vi "Key.vi"(6 "Scale":T1=enum."DO", 8 "Key":u8, 9 "Enable":bool) -> (0 "M":fxp<+,32,32>, 4 "Key out":u8)   [LabVIEW 2015]
uses:
  TypeDefs Host/Scales.ctl
panel:
  # "1"
  # "2"
  # "3"
  # "4"
  # "5"
  # "DO\nDO#\nRE\nRE#\nMI\nFA\nFA#\nSOL\nSOL#\nLA\nLA#\nSI"
  # "65,41\n69,30\n73,42\n77,78\n82,41\n87,31\n92,50\n98\n103,83\n110\n116,62\n123,47"
  # "130.82\n138.59\n146.83\n155.56\n164.81\n174.61\n185\n196\n207.65\n220\n233.08\n246.94"
  # "261.63\n277.18\n293.66\n311.13\n329.63\n349.23\n369.99\n392\n415.3\n440\n466.16\n493.88"
  # "523.25\n554.37\n587.33\n622.25\n659.26\n698.46\n739.99\n783.99\n830.61\n880\n932.33\n987.77"
  # "1046.5\n1108.73\n1174.66\n1244.51\n1318.51\n1396.91\n1479.98\n1567.98\n1661.22\n1760\n1864.66\n1975.53\n2093.00"
  # "65,41\n69,30\n73,42\n77,78\n82,41\n87,31\n92,50\n98\n103,83\n110\n116,62\n123,47"
  # "130.82\n138.59\n3941437,800448\n155.56\n4424084,750336\n174.61\n4966055,936\n5261334,9376\n207.65\n5905580,032\n233.08\n6628745,150464"
  # "261.63\n7440493,969408\n7882875,600896\n311.13\n8848437,936128\n349.23\n9931843,436544\n10522669,8752\n415.3\n11811160,064\n466.16\n13257490,300928"
  # "523.25\n14881256,374272\n15766019,637248\n622.25\n659.26\n698.46\n739.99\n783.99\n830.61\n880\n932.33\n987.77"
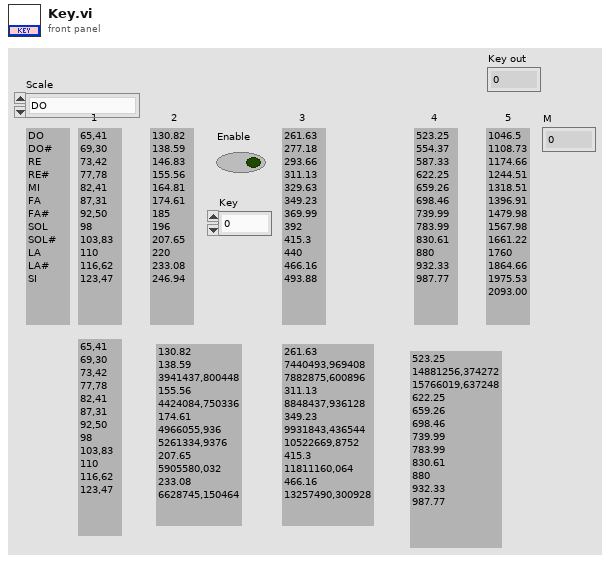
[diagram p1: front panel]
types:
  T1 = typedef "Scales.ctl" = enum16{"ALL", "DO", "RE"}
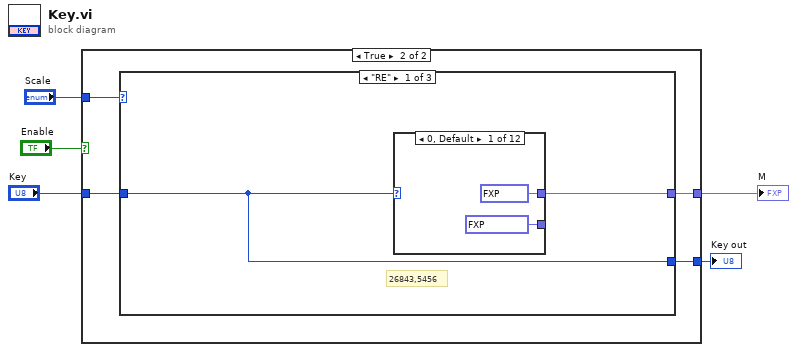
[diagram p0: block diagram]
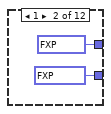
[diagram p3: hidden frame]
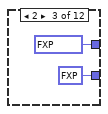
[diagram p4: hidden frame]
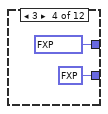
[diagram p5: hidden frame]
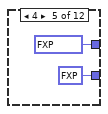
[diagram p6: hidden frame]
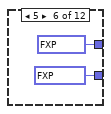
[diagram p7: hidden frame]
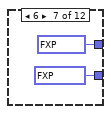
[diagram p8: hidden frame]
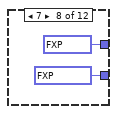
[diagram p9: hidden frame]
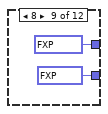
[diagram p10: hidden frame]
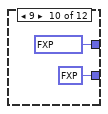
[diagram p11: hidden frame]
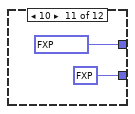
[diagram p12: hidden frame]
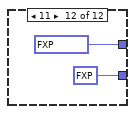
[diagram p13: hidden frame]
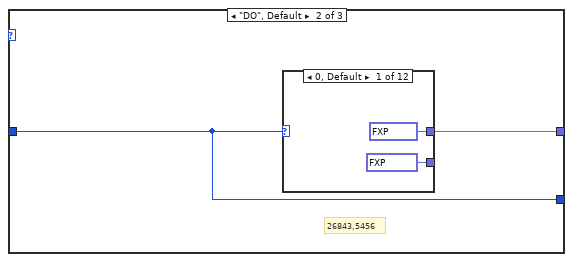
[diagram p14: hidden frame]
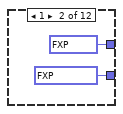
[diagram p15: hidden frame]
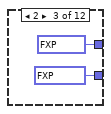
[diagram p16: hidden frame]
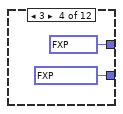
[diagram p17: hidden frame]
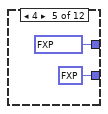
[diagram p18: hidden frame]
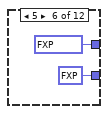
[diagram p19: hidden frame]
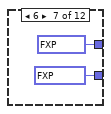
[diagram p20: hidden frame]
diagram:
  n1 = case shown="True" "Enable" {
    tunnel: "Key" -> [_ w9]
    tunnel: "Scale" -> [_ w8]
    tunnel: [_ w7] -> w3
    tunnel: [_ w6] -> w1
    frame False {
    }
    frame True {
      n2 = case shown="\"RE\"" w8 {
        tunnel: w9 -> [w10 w36 w65]
        tunnel: [w11 w37 w68] -> w7
        tunnel: [w10 w36 _] -> w6
        frame "RE" {
          # "26843,5456"
          n3 = case shown="0, Default" w10 {
            tunnel: [fxp<+,16,10> 146.828125 ("Fout 2") fxp<+,16,10> 164.8125 ("Fout 2") fxp<+,16,10> 185.0 ("Fout 2") fxp<+,16,10> 196.0 ("Fout 2") fxp<+,16,10> 220.0 ("Fout 2") fxp<+,16,10> 246.9375 ("Fout 2") fxp<+,16,10> 277.1875 ("Fout 2") fxp<+,16,10> 293.65625 ("Fout 2") fxp<+,16,10> 329.625 ("Fout 2") fxp<+,16,10> 370.0 ("Fout 2") fxp<+,16,10> 392.0 ("Fout 2") fxp<+,16,10> 440.0 ("Fout 2")] -> _
            tunnel: [fxp<+,32,32> 3941438.0 ("M 2") fxp<+,32,32> 4424085.0 ("M 2") fxp<+,32,32> 4966056.0 ("M 2") fxp<+,32,32> 5261335.0 ("M 2") fxp<+,32,32> 5905580.0 ("M 2") fxp<+,32,32> 6628745.0 ("M 2") fxp<+,32,32> 7440494.0 ("M 2") fxp<+,32,32> 7882876.0 ("M 2") fxp<+,32,32> 8848438.0 ("M 2") fxp<+,32,32> 9931843.0 ("M 2") fxp<+,32,32> 10522670.0 ("M 2") fxp<+,32,32> 11811160.0 ("M 2")] -> w11
            frame 0, Default {
            }
            frame 1 {
            }
            frame 2 {
            }
            frame 3 {
            }
            frame 4 {
            }
            frame 5 {
            }
            frame 6 {
            }
            frame 7 {
            }
            frame 8 {
            }
            frame 9 {
            }
            frame 10 {
            }
            frame 11 {
            }
          }
        }
        frame "DO", Default {
          # "26843,5456"
          n4 = case shown="0, Default" w36 {
            tunnel: [fxp<+,16,10> 130.8125 ("Fout 2") fxp<+,16,10> 146.828125 ("Fout 2") fxp<+,16,10> 164.8125 ("Fout 2") fxp<+,16,10> 174.609375 ("Fout 2") fxp<+,16,10> 196.0 ("Fout 2") fxp<+,16,10> 220.0 ("Fout 2") fxp<+,16,10> 246.9375 ("Fout 2") fxp<+,16,10> 261.625 ("Fout 2") fxp<+,16,10> 293.65625 ("Fout 2") fxp<+,16,10> 329.625 ("Fout 2") fxp<+,16,10> 349.234375 ("Fout 2") fxp<+,16,10> 392.0 ("Fout 2")] -> _
            tunnel: [fxp<+,32,32> 3511673.0 ("M 2") fxp<+,32,32> 3941438.0 ("M 2") fxp<+,32,32> 4424085.0 ("M 2") fxp<+,32,32> 4687151.0 ("M 2") fxp<+,32,32> 5261335.0 ("M 2") fxp<+,32,32> 5905580.0 ("M 2") fxp<+,32,32> 6628745.0 ("M 2") fxp<+,32,32> 7023077.0 ("M 2") fxp<+,32,32> 7882876.0 ("M 2") fxp<+,32,32> 8848438.0 ("M 2") fxp<+,32,32> 9374571.0 ("M 2") fxp<+,32,32> 10522670.0 ("M 2")] -> w37
            frame 0, Default {
            }
            frame 1 {
            }
            frame 2 {
            }
            frame 3 {
            }
            frame 4 {
            }
            frame 5 {
            }
            frame 6 {
            }
            frame 7 {
            }
            frame 8 {
            }
            frame 9 {
            }
            frame 10 {
            }
            frame 11 {
            }
          }
        }
        frame "ALL" {
          w66 = u8 24 ("y")
          w77 = u8 12 ("y")
          # "26843,5456"
          n5 = Subtract(x=w65, y=w77) -> (x-y=w76:u8)
          n6 = Greater Or Equal?(x=w65, y=w77) -> (x >= y?=w75:bool)
          n7 = Greater Or Equal?(x=w65, y=w66) -> (x >= y?=w67:bool)
          n8 = Subtract(x=w65, y=w66) -> (x-y=w64:u8)
          n9 = Select(t=w76, s=w75, f=w65) -> (s? t:f=w63:u8)
          n10 = Select(t=w64, s=w67, f=w63) -> (s? t:f=w62:u8)
          n11 = case shown="11" w62 {
            tunnel: [fxp<+,16,10> 130.8125 ("Fout 2") fxp<+,16,10> 138.59375 ("Fout 2") fxp<+,16,10> 146.828125 ("Fout 2") fxp<+,16,10> 155.5625 ("Fout 2") fxp<+,16,10> 164.8125 ("Fout 2") fxp<+,16,10> 174.609375 ("Fout 2") fxp<+,16,10> 185.0 ("Fout 2") fxp<+,16,10> 196.0 ("Fout 2") fxp<+,16,10> 207.65625 ("Fout 2") fxp<+,16,10> 220.0 ("Fout 2") fxp<+,16,10> 233.078125 ("Fout 2") fxp<+,16,10> 246.9375 ("Fout 2")] -> _
            tunnel: [fxp<+,32,32> 3511673.0 ("M 2") fxp<+,32,32> 3720247.0 ("M 2") fxp<+,32,32> 3941438.0 ("M 2") fxp<+,32,32> 4175782.0 ("M 2") fxp<+,32,32> 4424085.0 ("M 2") fxp<+,32,32> 4687151.0 ("M 2") fxp<+,32,32> 4966056.0 ("M 2") fxp<+,32,32> 5261335.0 ("M 2") fxp<+,32,32> 5574062.0 ("M 2") fxp<+,32,32> 5905580.0 ("M 2") fxp<+,32,32> 6256694.0 ("M 2") fxp<+,32,32> 6628745.0 ("M 2")] -> w70
            frame 0, Default {
            }
            frame 1 {
            }
            frame 2 {
            }
            frame 3 {
            }
            frame 4 {
            }
            frame 5 {
            }
            frame 6 {
            }
            frame 7 {
            }
            frame 8 {
            }
            frame 9 {
            }
            frame 10 {
            }
            frame 11 {
            }
          }
          n12 = Scale By Power Of 2(n=i16 1, x=w70) -> (x*2^n=w74:fxp<+,32,32>)
          n13 = Scale By Power Of 2(n=i16 2, x=w70) -> (x*2^n=w69:fxp<+,32,32>)
          n14 = Select(t=w74, s=w75, f=w70) -> (s? t:f=w72:fxp<+,32,32>)
          n15 = Select(t=w69, s=w67, f=w72) -> (s? t:f=w68:fxp<+,32,32>)
        }
      }
    }
  }
  "M" <- w3
  "Key out" <- w1
